vi "Export - Tx Packet.vi"(8 "error in (no error)":errorcluster, 11 "Device Item Ref in":T12 format="%.0x") -> (0 "error out":errorcluster, 3 "Tx Packet":T1 {"threadOptions"."pclDecimation" max=16 step=1; "threadOptions"."loopPeriod" max=16 step=1; "threadOptions"."targetPriority" min=-2 max=16 step=1; "threadOptions"."targetProcessor" min=-2 max=16 step=1; "Endianness" items=["big-endian"=0, "little-endian"=2]})   [LabVIEW 2016, in "UDP-Custom-Device System Explorer.lvlib"]
uses:
  UDP-Custom-Device System Explorer.lvlib
  <vilib>/NI Veristand/Custom Device API/Custom Device Item Ref.ctl
  Types/XML - New/ImpExp - Tx Packet Data.ctl
  <vilib>/NI Veristand/Custom Device API/Custom Device Item Info.ctl
  Shared/Types/Shared - Channel Data Type.ctl
  Shared/Types/Shared - Buffered.PacketInfo.ctl
  Shared/Types/Shared - Pointer Encoding.ctl
  Shared/Types/Shared - Receive Buffer Options.ctl
  Shared/Types/Shared - Transmit Buffer Options.ctl
  Shared/Types/Shared - Transmit Flag Options.ctl
  Shared/Types/Shared - Transmit Echo Options.ctl
  Types/Threading/Thread Configuration.ctl
  Types/Threading/Thread Sync Reference.ctl
  Property Accessors/Shared Packet Accessors.lvlib
  Property Accessors/Tx Packet Accessors.lvlib
  <vilib>/NI VeriStand/Custom Device API/Custom Device API.lvlib
  Shared/UDP-Custom-Device Shared.lvlib
  <vilib>/NI VeriStand/Custom Device Tools/Custom Device Utility Library/Custom Device Utility Library.lvlib
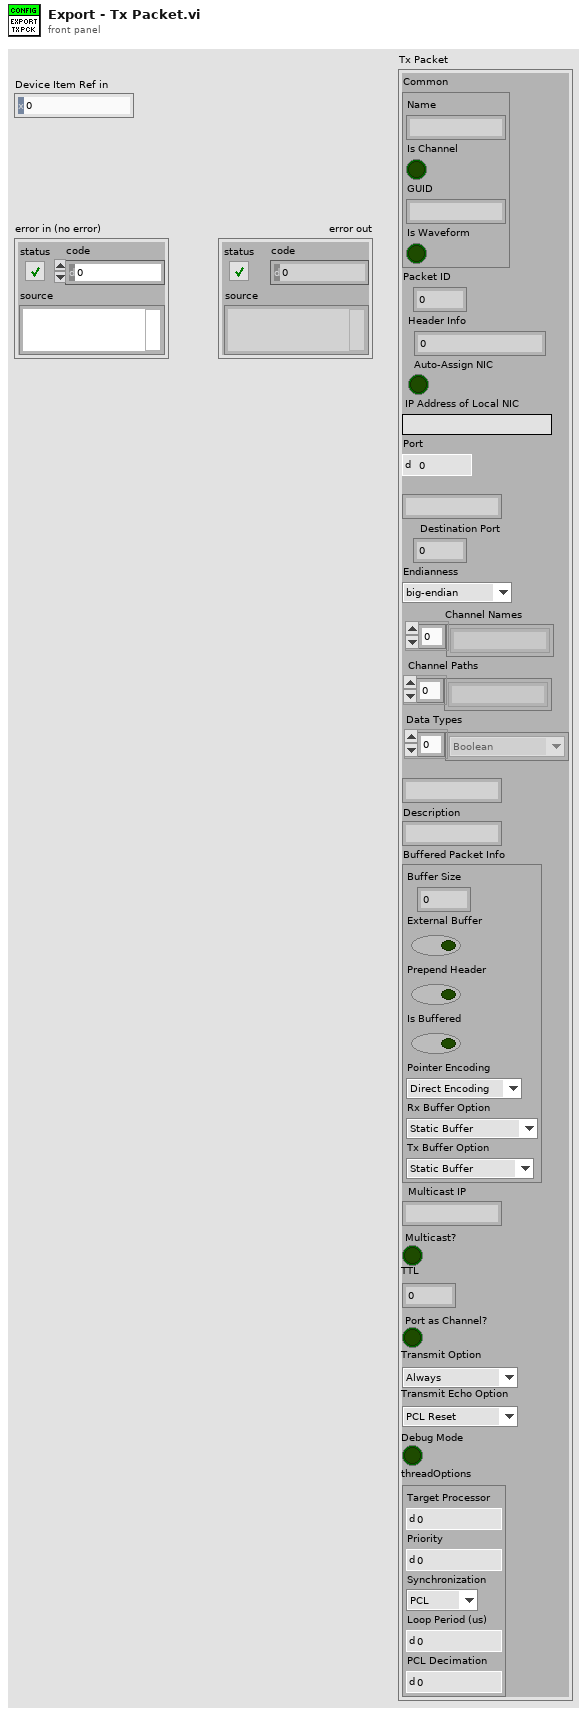
[diagram p1: front panel]
types:
  T1 = typedef "UDP-Custom-Device System Explorer.lvlib/ImpExp - Tx Packet Data.ctl" = cluster{"Common":T2, "Packet ID":i32, "Header Info":u32, "Auto-Assign NIC":bool, "IP Address of Local NIC":string, "Port":u16, "Destination IP":string, "Destination Port":u16, "Endianness":u16, "Channel Names":string[], "Channel Paths":string[], "Data Types":T3[], "Timestamp Path":string, "Description":string, "Buffered Packet Info":T4, "Multicast IP":string, "Multicast?":bool, "TTL":u16, "Port as Channel?":bool, "Transmit Option":T8, "Transmit Echo Option":T9, "Debug Mode":bool, "threadOptions":T10}
  T2 = typedef "Custom Device API.lvlib/Custom Device Item Info.ctl" = cluster{"Name":string, "Is Channel":bool, "GUID":string, "Is Waveform":bool}
  T3 = typedef "UDP-Custom-Device Shared.lvlib/Shared - Channel Data Type.ctl" = enum16{"Boolean", "Single", "Double", "I8", "I16", "I32", "I64", "U8", "U16", "U32", "U64"}
  T4 = typedef "UDP-Custom-Device Shared.lvlib/Shared - Buffered.PacketInfo.ctl" = cluster{"Buffer Size":i32, "External Buffer":bool, "Prepend Header":bool, "Is Buffered":bool, "Pointer Encoding":T5, "Rx Buffer Option":T6, "Tx Buffer Option":T7}
  T5 = typedef "UDP-Custom-Device Shared.lvlib/Shared - Pointer Encoding.ctl" = enum16{"Direct Encoding", "Conversion Encoding"}
  T6 = typedef "UDP-Custom-Device Shared.lvlib/Shared - Receive Buffer Options.ctl" = enum16{"Static Buffer", "Circular Buffer", "Circular Buffer + Size"}
  T7 = typedef "UDP-Custom-Device Shared.lvlib/Shared - Transmit Buffer Options.ctl" = enum16{"Static Buffer", "FIFO Buffer", "FIFO Buffer + Port"}
  T8 = typedef "UDP-Custom-Device Shared.lvlib/Shared - Transmit Flag Options.ctl" = enum16{"Always", "One-Shot", "Toggle"}
  T9 = typedef "UDP-Custom-Device Shared.lvlib/Shared - Transmit Echo Options.ctl" = enum16{"PCL Reset", "Counter", "Mirror"}
  T10 = typedef "UDP-Custom-Device System Explorer.lvlib/Thread Configuration.ctl" = cluster{"targetProcessor":i8, "targetPriority":i16, "Synchronization":T11, "loopPeriod":u32, "pclDecimation":u16}
  T11 = typedef "UDP-Custom-Device System Explorer.lvlib/Thread Sync Reference.ctl" = enum16{"PCL", "Async"}
  T12 = typedef "Custom Device API.lvlib/Custom Device Item Ref.ctl" = u64
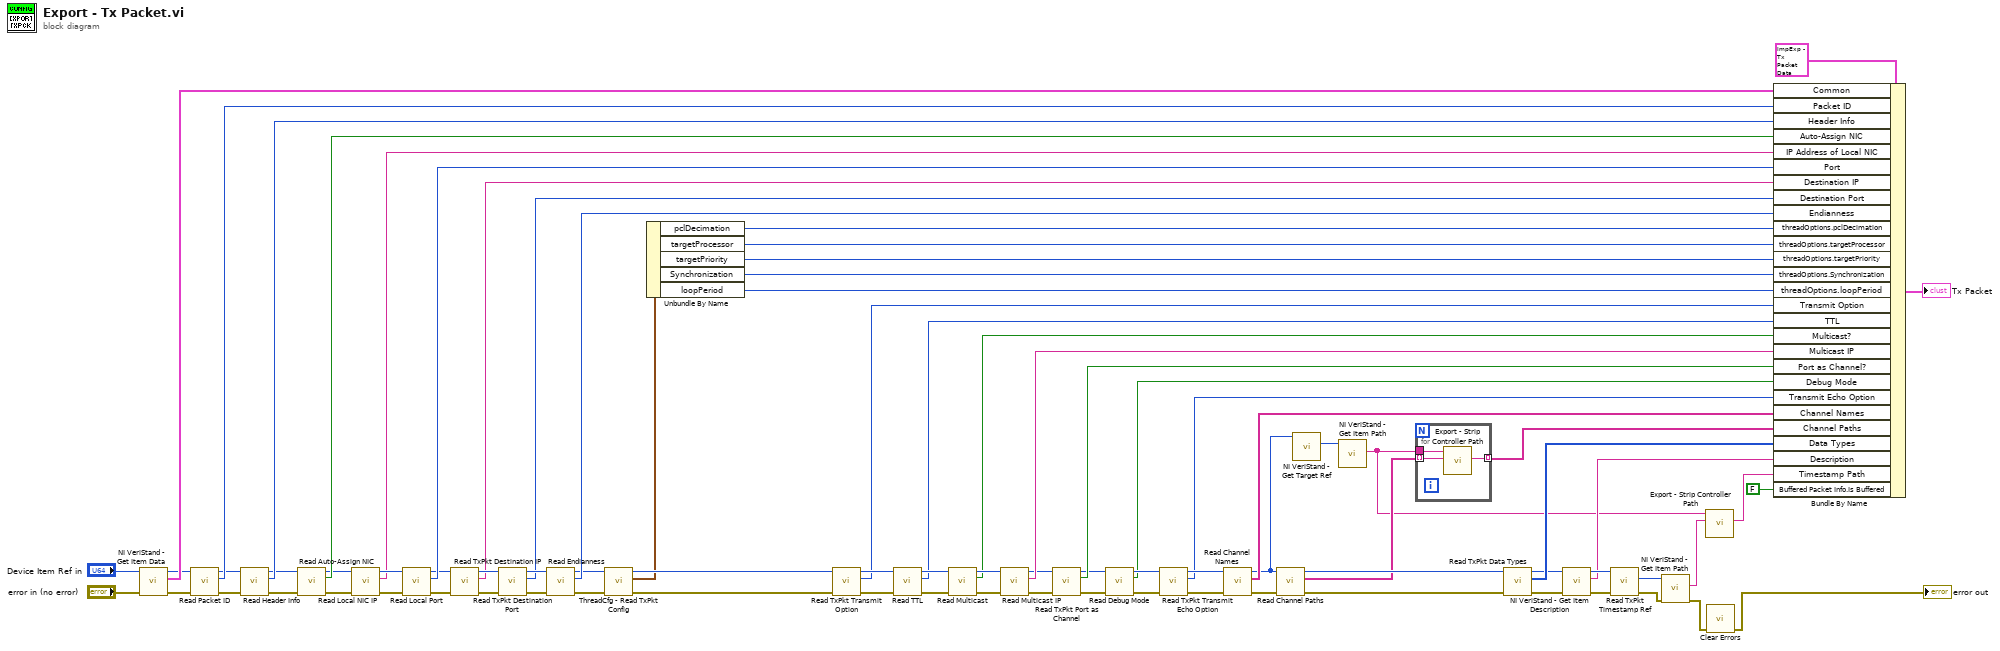
[diagram p0: block diagram]
diagram:
  n1 = call <vilib>:"NI VeriStand - Get Item Data.vi"("error in (no error)"="error in (no error)", "Item Ref in"="Device Item Ref in") -> ("error out"=w48:errorcluster, "Item Info"=w79:T2, "Item Ref out"=w78:T12)  [unwired: 6 in, 1 out]
  n2 = call "Read Packet ID.vi"("error in (no error)"=w48, "Node Ptr"=w78) -> ("error out"=w75:errorcluster, "Packet ID"=w77:i32, "Node Ptr out"=w76:T12)  [unwired: 7 in]
  n3 = call "Read Header Info.vi"("error in (no error)"=w75, "Node Ptr"=w76) -> ("error out"=w72:errorcluster, "Header Info"=w74:u32, "Node Ptr out"=w73:T12)  [unwired: 7 in]
  n4 = call "Read Auto-Assign NIC.vi"("error in (no error)"=w72, "Node Ptr"=w73) -> ("error out"=w67:errorcluster, "Auto-Assign NIC"=w71:bool, "Node Ptr out"=w70:T12)  [unwired: 7 in]
  n5 = call "Read Local NIC IP.vi"("error in (no error)"=w67, "Node Ptr"=w70) -> ("error out"=w68:errorcluster, "IP Address of Local NIC"=w66:string, "Node Ptr out"=w69:T12)  [unwired: 7 in]
  n6 = call "Read Local Port.vi"("error in (no error)"=w68, "Node Ptr"=w69) -> ("error out"=w63:errorcluster, "Port"=w65:u16, "Node Ptr out"=w64:T12)  [unwired: 7 in]
  n7 = call "Read TxPkt Destination IP.vi"("error in (no error)"=w63, "Node Ptr"=w64) -> ("error out"=w61:errorcluster, "Destination IP"=w58:string, "Node Ptr out"=w62:T12)  [unwired: 7 in]
  n8 = call "Read TxPkt Destination Port.vi"("error in (no error)"=w61, "Node Ptr"=w62) -> ("error out"=w59:errorcluster, "Destination Port"=w57:u16, "Node Ptr out"=w60:T12)  [unwired: 7 in]
  n9 = call "Read Endianness.vi"("error in (no error)"=w59, "Node Ptr"=w60) -> ("error out"=w7:errorcluster, "Endianness"=w56:u16, "Node Ptr out"=w8:T12)  [unwired: 7 in]
  n10 = call "ThreadCfg - Read TxPkt Config.vi"("error in (no error)"=w7, "Node Ptr In"=w8) -> ("error out"=w10:errorcluster, "threadOptions"=w6:T10, "Node Ptr Out"=w9:T12)  [unwired: 7 in]
  n11 = Unbundle By Name(w6) -> ("pclDecimation"=w5:u16, "targetProcessor"=w4:i8, "targetPriority"=w3:i16, "Synchronization"=w2:T11, "loopPeriod"=w1:u32)
  n12 = call "Read TxPkt Transmit Option.vi"("error in (no error)"=w10, "Node Ptr"=w9) -> ("error out"=w20:errorcluster, "Transmit Options"=w19:T8, "Node Ptr out"=w21:T12)  [unwired: 7 in]
  n13 = call "Read TTL.vi"("error in (no error)"=w20, "Node Ptr"=w21) -> ("error out"=w32:errorcluster, "TTL"=w28:u16, "Node Ptr out"=w31:T12)  [unwired: 7 in]
  n14 = call "Read Multicast.vi"("error in (no error)"=w32, "Node Ptr"=w31) -> ("error out"=w29:errorcluster, "Multicast"=w27:bool, "Node Ptr out"=w30:T12)  [unwired: 7 in]
  n15 = call "Read Multicast IP.vi"("error in (no error)"=w29, "Node Ptr"=w30) -> ("error out"=w23:errorcluster, "Multicast IP Address"=w26:string, "Node Ptr out"=w24:T12)  [unwired: 7 in]
  n16 = call "Read TxPkt Port as Channel.vi"("error in (no error)"=w23, "Node Ptr"=w24) -> ("error out"=w13:errorcluster, "Port as Channel"=w22:bool, "Node Ptr out"=w15:T12)  [unwired: 7 in]
  n17 = call "Read Debug Mode.vi"("error in (no error)"=w13, "Node Ptr"=w15) -> ("error out"=w12:errorcluster, "Debug Mode"=w11:bool, "Node Ptr out"=w14:T12)  [unwired: 7 in]
  n18 = call "Read TxPkt Transmit Echo Option.vi"("error in (no error)"=w12, "Node Ptr"=w14) -> ("error out"=w18:errorcluster, "Transmit Echo Options"=w16:T9, "Node Ptr out"=w17:T12)  [unwired: 7 in]
  n19 = call "Read Channel Names.vi"("error in (no error)"=w18, "Node Ptr"=w17) -> ("error out"=w55:errorcluster, "Channel Names"=w54:string[], "Node Ptr out"=w38:T12)  [unwired: 7 in]
  n20 = call "Read Channel Paths.vi"("error in (no error)"=w55, "Node Ptr"=w38) -> ("error out"=w52:errorcluster, "Channel Paths"=w37:string[], "Node Ptr out"=w53:T12)  [unwired: 7 in]
  n21 = call <vilib>:"NI VeriStand - Get Target Ref.vi"("Item Ref in"=w38) -> ("Target Ref"=w39:T12)  [unwired: 7 in, 3 out]
  n22 = call <vilib>:"NI VeriStand - Get Item Path.vi"("Item Ref in"=w39) -> ("Path"=w35:string)  [unwired: 7 in, 3 out]
  n23 = for {
    tunnel: w37 -> [w85] mode=indexing
    tunnel: w35 -> [w84]
    tunnel: [w83] -> w36 mode=indexing
    n24 = call "Export - Strip Controller Path.vi"("Channel Path"=w85, "Controller Path"=w84) -> ("Stripped Path"=w83:string)  [unwired: 8 in, 1 out]
  }
  n25 = call "Read TxPkt Data Types.vi"("error in (no error)"=w52, "Node Ptr"=w53) -> ("error out"=w42:errorcluster, "Data types"=w51:T3[], "Node Ptr out"=w44:T12)  [unwired: 7 in]
  n26 = call <vilib>:"NI VeriStand - Get Item Description.vi"("error in (no error)"=w42, "Item Ref in"=w44) -> ("error out"=w41:errorcluster, "Description"=w40:string, "Item Ref out"=w43:T12)  [unwired: 6 in, 1 out]
  n27 = call "Read TxPkt Timestamp Ref.vi"("error in (no error)"=w41, "Node Ptr"=w43) -> ("error out"=w49:errorcluster, "Timestamp Ref"=w50:T12)  [unwired: 7 in, 1 out]
  n28 = call <vilib>:"NI VeriStand - Get Item Path.vi"("error in (no error)"=w49, "Item Ref in"=w50) -> ("error out"=w47:errorcluster, "Path"=w34:string)  [unwired: 6 in, 2 out]
  n29 = call "Export - Strip Controller Path.vi"("Channel Path"=w34, "Controller Path"=w35) -> ("Stripped Path"=w33:string)  [unwired: 8 in, 1 out]
  n30 = call <vilib>:"Clear Errors.vi"("error in (no error)"=w47) -> ("error out"=→"error out":errorcluster)  [unwired: 5 in, 1 out]
  n31 = Bundle By Name(cluster=T1 {"Common"={"Name"="", "Is Channel"=FALSE, "GUID"="", "Is Waveform"=FALSE}, "Packet ID"=0, "Header Info"=0, "Auto-Assign NIC"=FALSE, "IP Address of Local NIC"="", "Port"=0, "Destination IP"="", "Destination Port"=0, "Endianness"=0, "Channel Names"=[], "Channel Paths"=[], "Data Types"=[], "Timestamp Path"="", "Description"="", "Buffered Packet Info"={"Buffer Size"=0, "External Buffer"=FALSE, "Prepend Header"=FALSE, "Is Buffered"=FALSE, "Pointer Encoding"=enum."Direct Encoding", "Rx Buffer Option"=enum."Static Buffer", "Tx Buffer Option"=enum."Static Buffer"}, "Multicast IP"="", "Multicast?"=FALSE, "TTL"=0, "Port as Channel?"=FALSE, "Transmit Option"=enum."Always", "Transmit Echo Option"=enum."PCL Reset", "Debug Mode"=FALSE, "threadOptions"={"targetProcessor"=0, "targetPriority"=0, "Synchronization"=enum."PCL", "loopPeriod"=0, "pclDecimation"=0}} ("Tx Packet"), "Common"=w79, "Packet ID"=w77, "Header Info"=w74, "Auto-Assign NIC"=w71, "IP Address of Local NIC"=w66, "Port"=w65, "Destination IP"=w58, "Destination Port"=w57, "Endianness"=w56, "threadOptions.pclDecimation"=w5, "threadOptions.targetProcessor"=w4, "threadOptions.targetPriority"=w3, "threadOptions.Synchronization"=w2, "threadOptions.loopPeriod"=w1, "Transmit Option"=w19, "TTL"=w28, "Multicast?"=w27, "Multicast IP"=w26, "Port as Channel?"=w22, "Debug Mode"=w11, "Transmit Echo Option"=w16, "Channel Names"=w54, "Channel Paths"=w36, "Data Types"=w51, "Description"=w40, "Timestamp Path"=w33, "Buffered Packet Info.Is Buffered"=FALSE) -> (→"Tx Packet":T1)
